vi "Drive_Execute.vi"() -> ()   [LabVIEW 2020]
uses:
  Globals/Drive_Globals.vi
  Globals/Sensor_Values.vi
  Drive_Control_States.ctl
  Drive_Orientation_States.ctl
  Drive_Cluster.ctl
panel:
  out "angles":T1(graph)={"Front_Right"=164.54498291015625, "Front_ Left"=166.52252197265625, "Back_Left"=-15.897216796875, "Back_Right"=-14.60357666015625}
  out "Front_Right":T2(graph)={"Command"=0.0432740478515625, "Proportional"=0.0432740478515625, "Integral"=0.0, "Derivative"=0.0, "Goal"=15.45501708984375}
  out "Back_Right":T2(graph)={"Command"=0.0408900146484375, "Proportional"=0.0408900146484375, "Integral"=0.0, "Derivative"=0.0, "Goal"=14.60357666015625}
  out "Back_Left":T2(graph)={"Command"=0.04451220703125, "Proportional"=0.04451220703125, "Integral"=0.0, "Derivative"=0.0, "Goal"=15.897216796875}
  out "Front_Left":T2(graph)={"Command"=0.0377369384765625, "Proportional"=0.0377369384765625, "Integral"=0.0, "Derivative"=0.0, "Goal"=13.47747802734375}
  in  "Manual_Target_Angle (deg)":dbl
  in  "Front_Panel_Control":bool
  in  "Hysteresis (deg)":dbl=10.0 format="%#_13g"
  in  "Back_Right_PID":T3={"Kp"=0.0028, "Ki"=0.0, "Kd"=0.0, "N-Diff"=10, "N-Int"=10, "Int Error Window"=20.0, "Max Ouput"=0.5, "Min Output"=-0.5} {"Int Error Window" min=0.0; "N-Int" min=2; "N-Diff" min=2; "Kd" min=0.0; "Ki" min=0.0; "Kp" min=0.0}
  in  "Back_Left_PID":T3={"Kp"=0.0028, "Ki"=0.0, "Kd"=0.0, "N-Diff"=10, "N-Int"=10, "Int Error Window"=20.0, "Max Ouput"=0.5, "Min Output"=-0.5} {"Int Error Window" min=0.0; "N-Int" min=2; "N-Diff" min=2; "Kd" min=0.0; "Ki" min=0.0; "Kp" min=0.0}
  in  "Front_Left_PID":T3={"Kp"=0.0028, "Ki"=0.0, "Kd"=0.0, "N-Diff"=10, "N-Int"=10, "Int Error Window"=20.0, "Max Ouput"=0.5, "Min Output"=-0.5} {"Int Error Window" min=0.0; "N-Int" min=2; "N-Diff" min=2; "Kd" min=0.0; "Ki" min=0.0; "Kp" min=0.0}
  in  "Front_Right_PID":T3={"Kp"=0.0028, "Ki"=0.0, "Kd"=0.0, "N-Diff"=10, "N-Int"=10, "Int Error Window"=20.0, "Max Ouput"=0.5, "Min Output"=-0.5} {"Int Error Window" min=0.0; "N-Int" min=2; "N-Diff" min=2; "Kd" min=0.0; "Ki" min=0.0; "Kp" min=0.0}
  # ".0025"
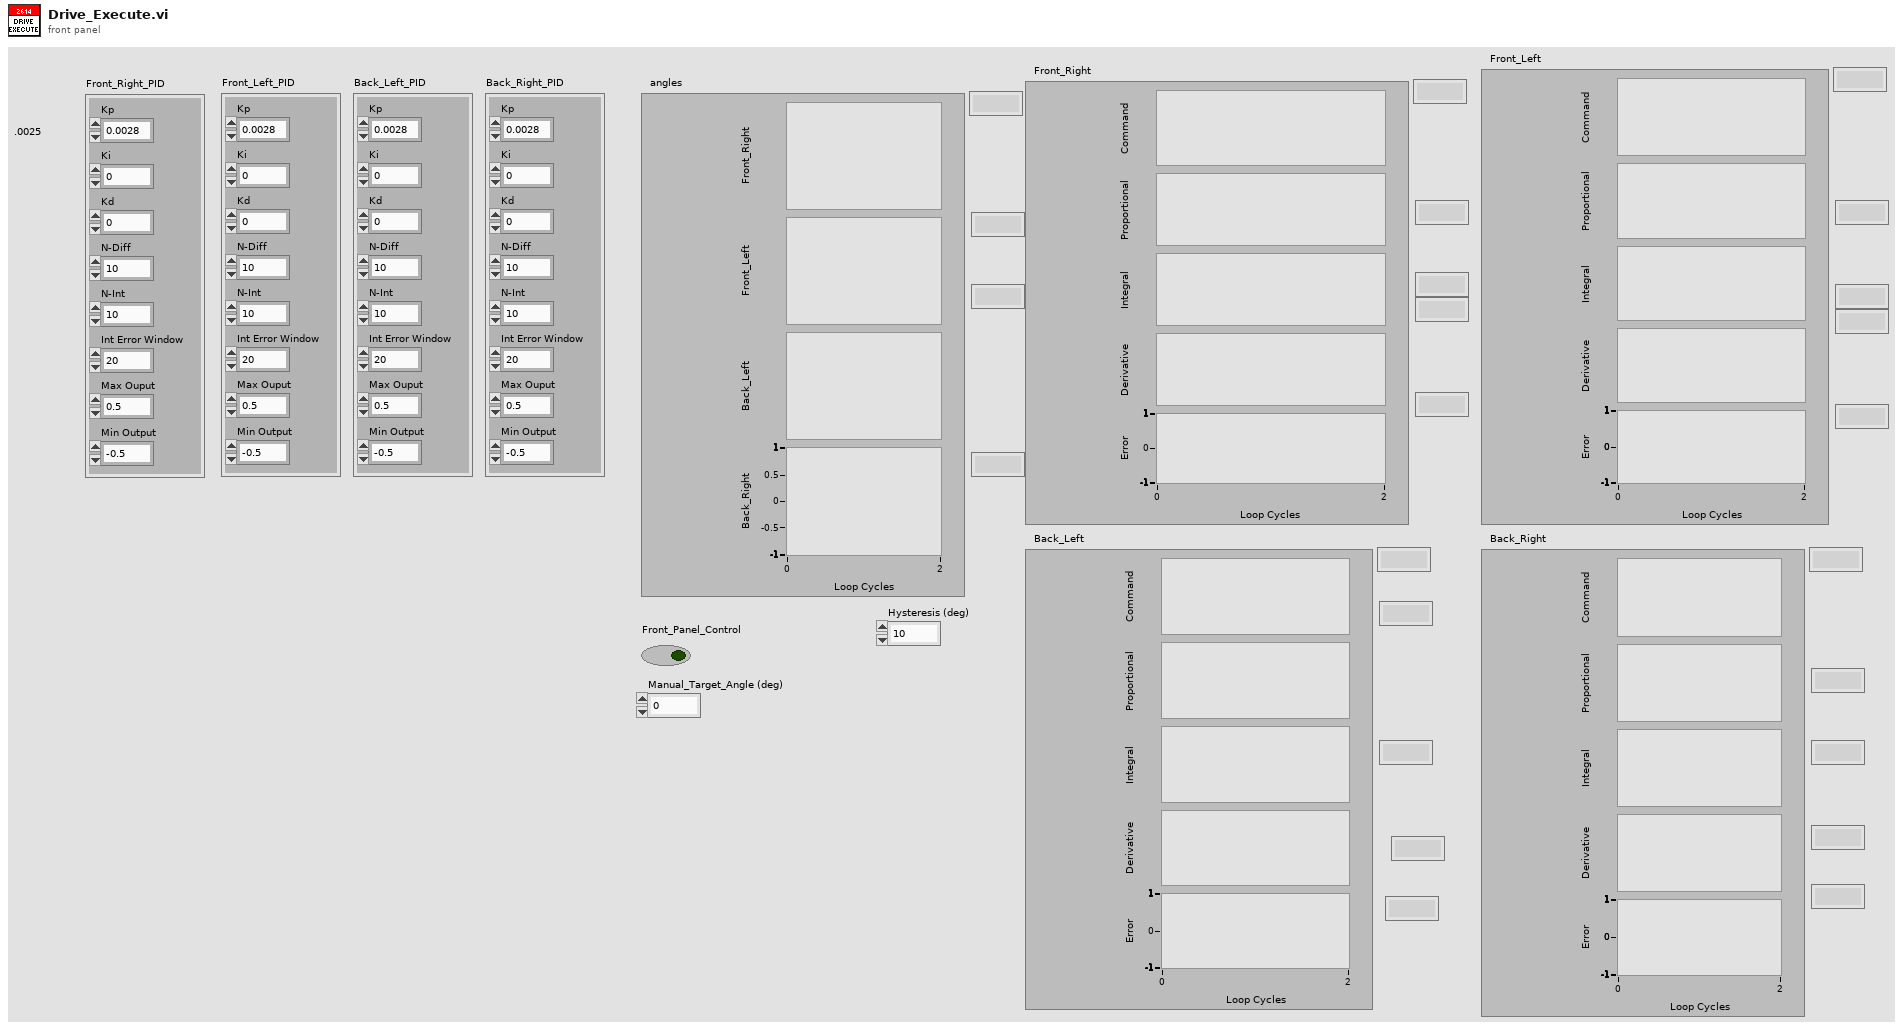
[diagram p1: front panel]
types:
  T1 = cluster{"Front_Right":dbl, "Front_ Left":dbl, "Back_Left":dbl, "Back_Right":dbl}
  T2 = cluster{"Command":dbl, "Proportional":dbl, "Integral":dbl, "Derivative":dbl, "Goal":dbl}
  T3 = cluster{"Kp":dbl, "Ki":dbl, "Kd":dbl, "N-Diff":i32, "N-Int":i32, "Int Error Window":dbl, "Max Ouput":dbl, "Min Output":dbl}
  T4 = typedef "Drive_Control_States.ctl" = enum16{"No-Op", "Manual_Control", "Command_DriveDistanceAtAngle", "Command_DrivePath", "Command_SetRobotPose"}
  T5 = typedef "Drive_Cluster.ctl" = cluster{"Control_State":T4, "Vertical_Throttle":dbl, "Lateral_Throttle":dbl, "Rotational_Throttle":dbl, "Strafe_In_Deadband":bool, "Rotation_In_Deadband":bool, "Orientation_State":T6, "Parameters":dbl[], "Step":i32, "Auto_Notifier":refnum<notifier>, "PathName":string}
  T6 = typedef "Drive_Orientation_States.ctl" = enum16{"Robot-Oriented", "Field-Oriented"}
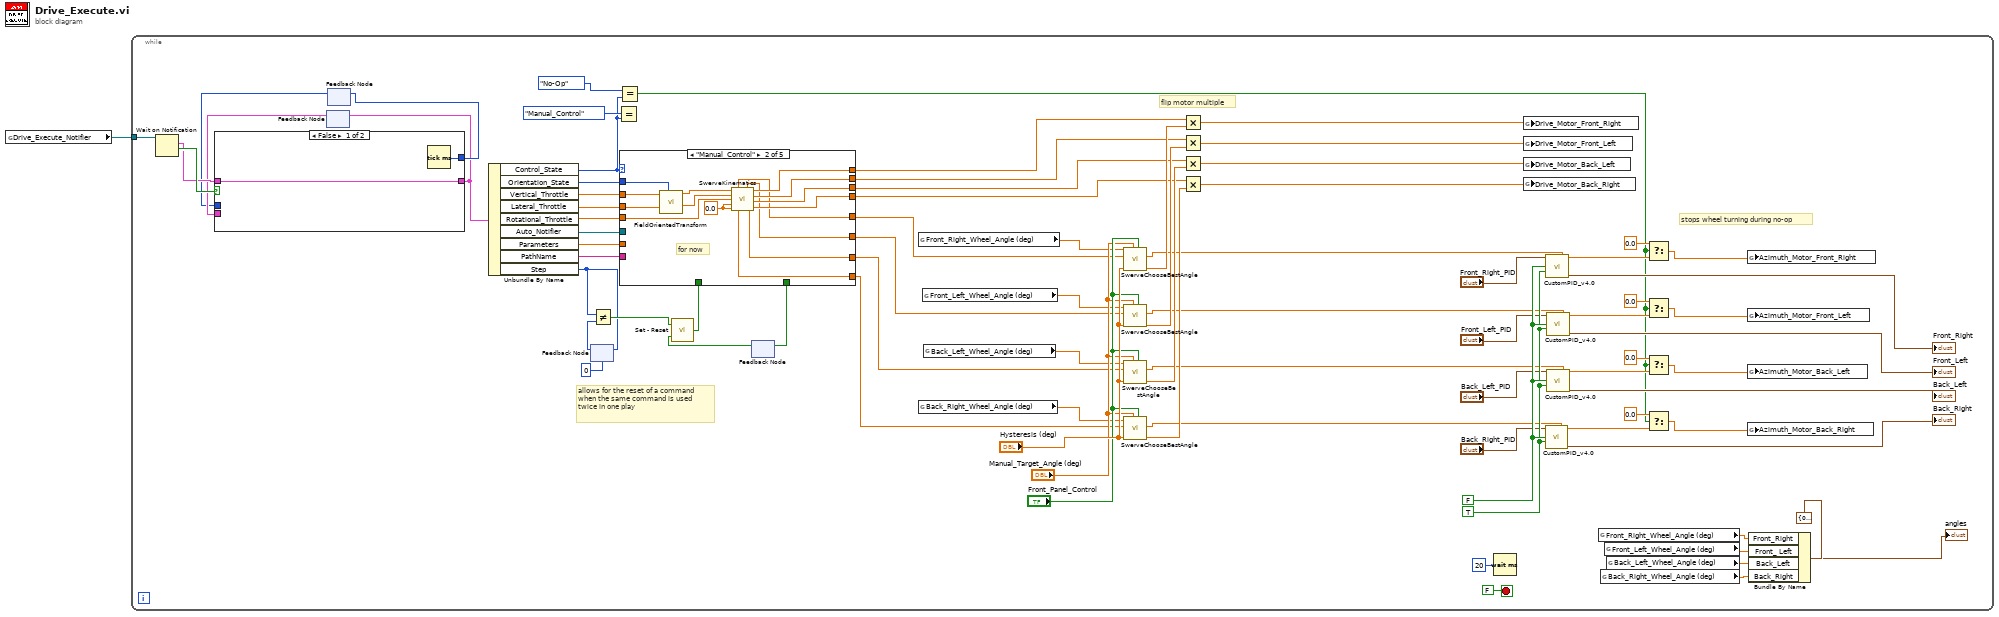
[diagram p0: block diagram]
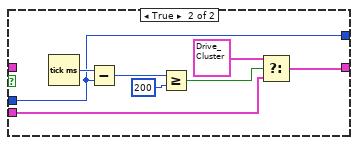
[diagram p2: hidden frame]
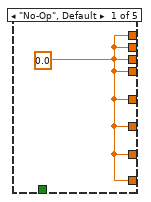
[diagram p3: hidden frame]
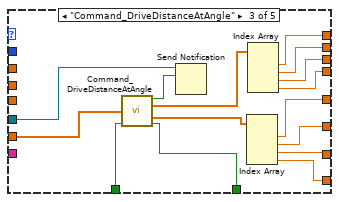
[diagram p4: hidden frame]
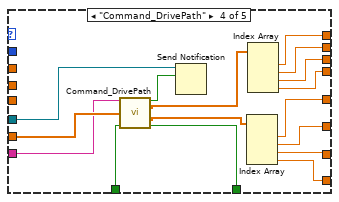
[diagram p5: hidden frame]
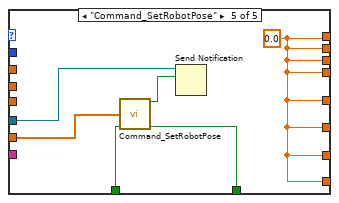
[diagram p6: hidden frame]
diagram:
  n1 = global read "Drive_Globals.vi" "Drive_Execute_Notifier"() -> (w1:refnum<notifier>)
  n2 = while {
    tunnel: w1 -> [w81]
    stop <- FALSE stop-if-true
    w78 = TRUE
    w79 = FALSE
    # "stops wheel turning during no-op"
    # "flip motor multiple"
    # "allows for the reset of a command when the same command is used twice in one play"
    n3 = Wait on Notification(notifier=w81) -> (notification=w18:T5, timed out?=w19:bool)  [unwired: 3 in, 2 out]
    n4 = feedback #1() -> (w17:T5)  [unwired: 1 in]
    n5 = feedback #2() -> (w15:u32)  [unwired: 1 in]
    n6 = case shown="False" w19 {
      tunnel: w18 -> [w85 _]
      tunnel: [w85 w93] -> w14
      tunnel: w17 -> [_ w92]
      tunnel: [w84 w90] -> w16
      tunnel: w15 -> [_ w90]
      frame False {
        n7 = Tick Count (ms)() -> (millisecond timer value=w84:u32)
      }
      frame True {
        n8 = Tick Count (ms)() -> (millisecond timer value=w91:u32)
        n9 = Subtract(x=w91, y=w90) -> (x-y=w88:u32)
        n10 = Greater Or Equal?(x=w88, y=u32 200) -> (x >= y?=w89:bool)
        n11 = Select(t=T5 {"Control_State"=enum."Manual_Control", "Vertical_Throttle"=0.0, "Lateral_Throttle"=0.0, "Rotational_Throttle"=0.0, "Strafe_In_Deadband"=FALSE, "Rotation_In_Deadband"=FALSE, "Orientation_State"=enum."Robot-Oriented", "Parameters"=[], "Step"=0, "Auto_Notifier"=refnum, "PathName"=""} ("Cluster"), s=w89, f=w92) -> (s? t:f=w93:T5)
      }
    }
    n12 = feedback-in #1(w14) -> ()
    n13 = feedback-in #2(w16) -> ()
    n14 = Unbundle By Name(w14) -> ("Control_State"=w8:T4, "Orientation_State"=w80:T6, "Vertical_Throttle"=w65:dbl, "Lateral_Throttle"=w64:dbl, "Rotational_Throttle"=w72:dbl, "Auto_Notifier"=w54:refnum<notifier>, "Parameters"=w53:dbl[], "PathName"=w2:string, "Step"=w3:i32)
    n15 = feedback-in #3(w3) -> ()
    n16 = feedback #3(0 ("Step")) -> (w52:i32)
    n17 = Not Equal?(x=w3, y=w52) -> (x != y?=w12:bool)
    n18 = Equal?(x=Drive_Control_States."Manual_Control" ("Control_State"), y=w8) -> ()  [unwired: 1 out]
    n19 = Equal?(x=Drive_Control_States."No-Op", y=w8) -> (x = y?=w25:bool)
    n20 = feedback #4() -> (w11:bool)  [unwired: 1 in]
    n21 = call "Set - Reset.vi"("Reset"=w11, "Set"=w12) -> ("Output"=w10:bool)
    n22 = case shown="\"Manual_Control\"" w8 {
      tunnel: [w94 w105 w120 w139 w141] -> w41
      tunnel: [w94 w104 w119 w138 w141] -> w40
      tunnel: [w94 w103 w118 w137 w141] -> w39
      tunnel: [w94 w102 w117 w136 w141] -> w38
      tunnel: [w94 w101 w115 w135 w141] -> w49
      tunnel: [w94 w100 w114 w134 w141] -> w48
      tunnel: [w94 w99 w113 w133 w141] -> w47
      tunnel: [w94 w98 w112 w132 w141] -> w46
      tunnel: w72 -> [_ w107 _ _ _]
      tunnel: w80 -> [_ w95 _ _ _]
      tunnel: w65 -> [_ w96 _ _ _]
      tunnel: w64 -> [_ w97 _ _ _]
      tunnel: w54 -> [_ _ w123 w140 w146]
      tunnel: w53 -> [_ _ w124 w130 w144]
      tunnel: w10 -> [_ _ w111 w131 w145]
      tunnel: [_ _ w110 w126 w142] -> w13
      tunnel: w2 -> [_ _ _ w125 _]
      frame "No-Op", Default {
        w94 = 0.0 ("Numeric")
      }
      frame "Manual_Control" {
        w106 = 0.0 ("Cx (in)")
        # "for now"
        n23 = call "FieldOrientedTransform.vi"("Orientation Mode"=w95, "Joystick Y"=w97, "Joystick X"=w96) -> ("Joystick Y'"=w108:dbl, "Joystick X'"=w109:dbl)  [unwired: 7 in]
        n24 = call "SwerveKinematics.vi"("Joystick X"=w109, "Joystick Y"=w108, "Joystick Rotation"=w107, "Cx (in)"=w106, "Cy (in)"=w106) -> ("Module 0 Angle (deg)"=w101:dbl, "Module 1 Angle (deg)"=w100:dbl, "Module 0 Velocity Command (ul)"=w105:dbl, "Module 1 Velocity Command (ul)"=w104:dbl, "Module 2 Velocity Command (ul)"=w103:dbl, "Module 3 Angle (deg)"=w98:dbl, "Module 2 Angle (deg)"=w99:dbl, "Module 3 Velocity Command (ul)"=w102:dbl)  [unwired: 3 in]
      }
      frame "Command_DriveDistanceAtAngle" {
        n25 = call "Command_DriveDistanceAtAngle.vi"("Parameters"=w124, "Startup"=w111) -> ("Completed"=w122:bool, "Target_Drive_Powers"=w121:dbl[], "Target_Wheel_Angles"=w116:dbl[], "Reinit"=w110:bool)  [unwired: 10 in]
        n26 = Send Notification(notification=w122, notifier=w123) -> ()  [unwired: 1 in, 2 out]
        n27 = Index Array(array=w116) -> (element #1=w115:dbl, element #2=w114:dbl, element #3=w113:dbl, element #4=w112:dbl)  [unwired: 4 in]
        n28 = Index Array(array=w121) -> (element #1=w120:dbl, element #2=w119:dbl, element #3=w118:dbl, element #4=w117:dbl)  [unwired: 4 in]
      }
      frame "Command_DrivePath" {
        n29 = call "Command_DrivePath.vi"("Name of Path"=w125, "Parameters"=w130, "Startup"=w131) -> ("Completed"=w127:bool, "Drive_Motor_Values"=w129:dbl[], "Azimuth_Motor_Values"=w128:dbl[], "Reinit"=w126:bool)  [unwired: 9 in]
        n30 = Send Notification(notification=w127, notifier=w140) -> ()  [unwired: 1 in, 2 out]
        n31 = Index Array(array=w128) -> (element #1=w135:dbl, element #2=w134:dbl, element #3=w133:dbl, element #4=w132:dbl)  [unwired: 4 in]
        n32 = Index Array(array=w129) -> (element #1=w139:dbl, element #2=w138:dbl, element #3=w137:dbl, element #4=w136:dbl)  [unwired: 4 in]
      }
      frame "Command_SetRobotPose" {
        w141 = 0.0 ("Numeric")
        n33 = call "Command_SetRobotPose.vi"("Parameters"=w144, "Startup"=w145) -> ("Completed"=w143:bool, "Reinit"=w142:bool)  [unwired: 12 in]
        n34 = Send Notification(notification=w143, notifier=w146) -> ()  [unwired: 1 in, 2 out]
      }
    }
    n35 = feedback-in #4(w13) -> ()
    n36 = global read "Sensor_Values.vi" "Front_Right_Wheel_Angle (deg)"() -> (w50:dbl)
    n37 = global read "Sensor_Values.vi" "Back_Right_Wheel_Angle (deg)"() -> (w59:dbl)
    n38 = global read "Sensor_Values.vi" "Front_Left_Wheel_Angle (deg)"() -> (w61:dbl)
    n39 = global read "Sensor_Values.vi" "Back_Left_Wheel_Angle (deg)"() -> (w60:dbl)
    n40 = call "SwerveChooseBestAngle.vi"("Goal Override"="Front_Panel_Control", "Goal Override Angle (deg) [-180,+180]"="Manual_Target_Angle (deg)", "Hysteresis (deg)"="Hysteresis (deg)", "Goal Angle (deg) [-180,+180]"=w49, "Current Angle (deg) [-180,+180]"=w50) -> ("Flip Drive Motor Multiple"=w76:dbl, "Angular Distance (deg)"=w7:dbl)  [unwired: 5 in]
    n41 = call "SwerveChooseBestAngle.vi"("Goal Override"="Front_Panel_Control", "Goal Override Angle (deg) [-180,+180]"="Manual_Target_Angle (deg)", "Hysteresis (deg)"="Hysteresis (deg)", "Goal Angle (deg) [-180,+180]"=w48, "Current Angle (deg) [-180,+180]"=w61) -> ("Flip Drive Motor Multiple"=w75:dbl, "Angular Distance (deg)"=w6:dbl)  [unwired: 5 in]
    n42 = call "SwerveChooseBestAngle.vi"("Goal Override"="Front_Panel_Control", "Goal Override Angle (deg) [-180,+180]"="Manual_Target_Angle (deg)", "Hysteresis (deg)"="Hysteresis (deg)", "Goal Angle (deg) [-180,+180]"=w47, "Current Angle (deg) [-180,+180]"=w60) -> ("Flip Drive Motor Multiple"=w74:dbl, "Angular Distance (deg)"=w5:dbl)  [unwired: 5 in]
    n43 = call "SwerveChooseBestAngle.vi"("Goal Override"="Front_Panel_Control", "Goal Override Angle (deg) [-180,+180]"="Manual_Target_Angle (deg)", "Hysteresis (deg)"="Hysteresis (deg)", "Goal Angle (deg) [-180,+180]"=w46, "Current Angle (deg) [-180,+180]"=w59) -> ("Flip Drive Motor Multiple"=w73:dbl, "Angular Distance (deg)"=w4:dbl)  [unwired: 5 in]
    n44 = Multiply(x=w41, y=w76) -> (x*y=w37:dbl)
    n45 = Multiply(x=w40, y=w75) -> (x*y=w36:dbl)
    n46 = Multiply(x=w39, y=w74) -> (x*y=w35:dbl)
    n47 = Multiply(x=w38, y=w73) -> (x*y=w34:dbl)
    n48 = Wait (ms)(milliseconds to wait=u32 20) -> ()  [unwired: 1 out]
    n49 = global write "Drive_Globals.vi" "Drive_Motor_Front_Right"(w37) -> ()
    n50 = global write "Drive_Globals.vi" "Drive_Motor_Front_Left"(w36) -> ()
    n51 = global write "Drive_Globals.vi" "Drive_Motor_Back_Left"(w35) -> ()
    n52 = global write "Drive_Globals.vi" "Drive_Motor_Back_Right"(w34) -> ()
    n53 = call "CustomPID_v4.0.vi"("PID Tuning Parameters"="Back_Right_PID", "Custom Error Calculation"=w4, "Reset on Goal Change ?"=w79, "Use Custom Error Calculation ?"=w78) -> ("Command"=w33:dbl, "Controller Summary"=→"Back_Right":T2)  [unwired: 8 in, 2 out]
    n54 = call "CustomPID_v4.0.vi"("PID Tuning Parameters"="Front_Right_PID", "Custom Error Calculation"=w7, "Reset on Goal Change ?"=w79, "Use Custom Error Calculation ?"=w78) -> ("Command"=w26:dbl, "Controller Summary"=→"Front_Right":T2)  [unwired: 8 in, 2 out]
    n55 = call "CustomPID_v4.0.vi"("PID Tuning Parameters"="Front_Left_PID", "Custom Error Calculation"=w6, "Reset on Goal Change ?"=w79, "Use Custom Error Calculation ?"=w78) -> ("Command"=w27:dbl, "Controller Summary"=→"Front_Left":T2)  [unwired: 8 in, 2 out]
    n56 = call "CustomPID_v4.0.vi"("PID Tuning Parameters"="Back_Left_PID", "Custom Error Calculation"=w5, "Reset on Goal Change ?"=w79, "Use Custom Error Calculation ?"=w78) -> ("Command"=w28:dbl, "Controller Summary"=→"Back_Left":T2)  [unwired: 8 in, 2 out]
    n57 = global read "Sensor_Values.vi" "Front_Right_Wheel_Angle (deg)"() -> (w55:dbl)
    n58 = global read "Sensor_Values.vi" "Back_Right_Wheel_Angle (deg)"() -> (w56:dbl)
    n59 = global read "Sensor_Values.vi" "Front_Left_Wheel_Angle (deg)"() -> (w58:dbl)
    n60 = global read "Sensor_Values.vi" "Back_Left_Wheel_Angle (deg)"() -> (w57:dbl)
    n61 = Select(t=0.0, s=w25, f=w26) -> (s? t:f=w24:dbl)
    n62 = Select(t=0.0, s=w25, f=w27) -> (s? t:f=w23:dbl)
    n63 = Select(t=0.0, s=w25, f=w28) -> (s? t:f=w22:dbl)
    n64 = Select(t=0.0, s=w25, f=w33) -> (s? t:f=w21:dbl)
    n65 = global write "Drive_Globals.vi" "Azimuth_Motor_Front_Right"(w24) -> ()
    n66 = global write "Drive_Globals.vi" "Azimuth_Motor_Front_Left"(w23) -> ()
    n67 = global write "Drive_Globals.vi" "Azimuth_Motor_Back_Left"(w22) -> ()
    n68 = global write "Drive_Globals.vi" "Azimuth_Motor_Back_Right"(w21) -> ()
    n69 = Bundle By Name(cluster=T1 {"Front_Right"=0.0, "Front_ Left"=0.0, "Back_Left"=0.0, "Back_Right"=0.0}, "Front_Right"=w55, "Front_ Left"=w58, "Back_Left"=w57, "Back_Right"=w56) -> (→"angles":T1)
  }
